vi "setSession.vi"(8 "error in (no error)":errorcluster, 10 "Session":refnum<class "Session.Client.lvclass">, 11 "Client in":refnum<class "Client.lvclass">) -> (0 "error out":errorcluster, 3 "Client out":refnum<class "Client.lvclass">)   [LabVIEW 2013, in "MQTT Client.lvlib" / "Client.lvclass"]
uses:
  Client.lvclass
  Session.Client/Session.Client.lvclass
  Client.lvclass/Client.ctl
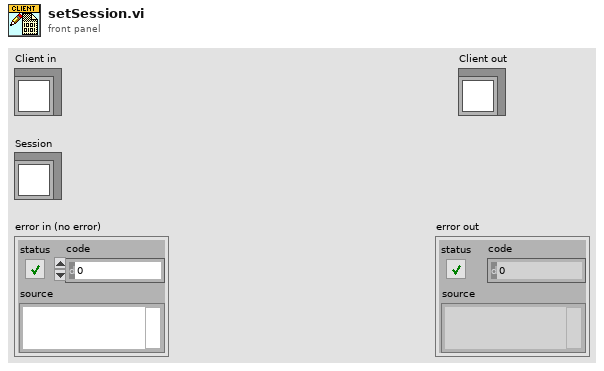
[diagram p1: front panel]
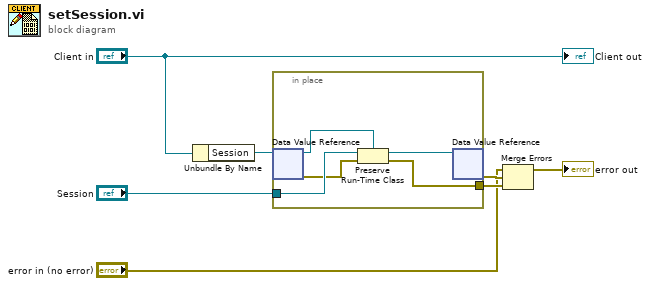
[diagram p0: block diagram]
diagram:
  n1 = Unbundle By Name("Client in") -> ("Session"=w6:refnum<data-value>)
  n2 = in-place {
    in-place-border: [w10] -> w4
    in-place-border: "Session" -> [w12]
    n3 = in-place-dvr #1(w6) -> (w8:refnum<class "Session.Client.lvclass">, w9:errorcluster)
    n4 = Preserve Run-Time Class(object in=w12, error in=w9, 2:w8) -> (object out=w11:refnum<class "Session.Client.lvclass">, error out=w10:errorcluster)
    n5 = in-place-dvr #1(w11) -> (w5:errorcluster)  [unwired: 1 out]
  }
  n6 = Merge Errors("error in (no error)", w5, w4) -> (→"error out":errorcluster)
  "Client out" <- "Client in"
